vi "Humidity_uncert_2024.vi"(0 "Temperature":dbl=293.15 format="%.4g", 1 "Temperature unit":i32(listbox), 4 "pressure unit":i32(listbox)=1, 5 "Pressure":dbl=100.0 format="%.3f", 6 "Humidity":dbl=50.0 format="%.6f", 7 "humidity unit":i32(listbox)=3) -> (3 "relative humidity":dbl=0.5 format="%.5f", 8 "Psat/p > 1/fe !":bool, 9 "Xw > 1 !":bool, 10 "saturation pressure / Pa":dbl=2339.2491605340156 format="%.1f", 11 "enhanc. factor":dbl=1.0035110316816116 format="%.5g", 12 "DPsat - saturation press. abs. uncert.":dbl=0.23392491605340157 format="%_3f", 13 "xw - molar fraction":dbl=0.011737311692239169, 14 "DPsat/Psat - saturation press. rel. uncert.":dbl=0.0001 format="%.1e", 15 "Def/ef - enhanc. fact. rel. uncert.":dbl=0.00045 format="%.1e", 16 "RH > 1 !":bool, 17 "Def - enhanc. fact. abs. uncert.":dbl=0.0004515799642567252 format="%.6f", 18 "Dxw - molar fraction abs. uncert.":dbl=6.455521430731544e-06 format="%.6f", 19 "Dxw/xw - molar fraction rel. uncert.":dbl=0.00055 format="%.1e")   [LabVIEW 2016]
panel:
  in  "Saturation below 273.16 K":i32(listbox)
  # "±"
  # "±"
  # "±"
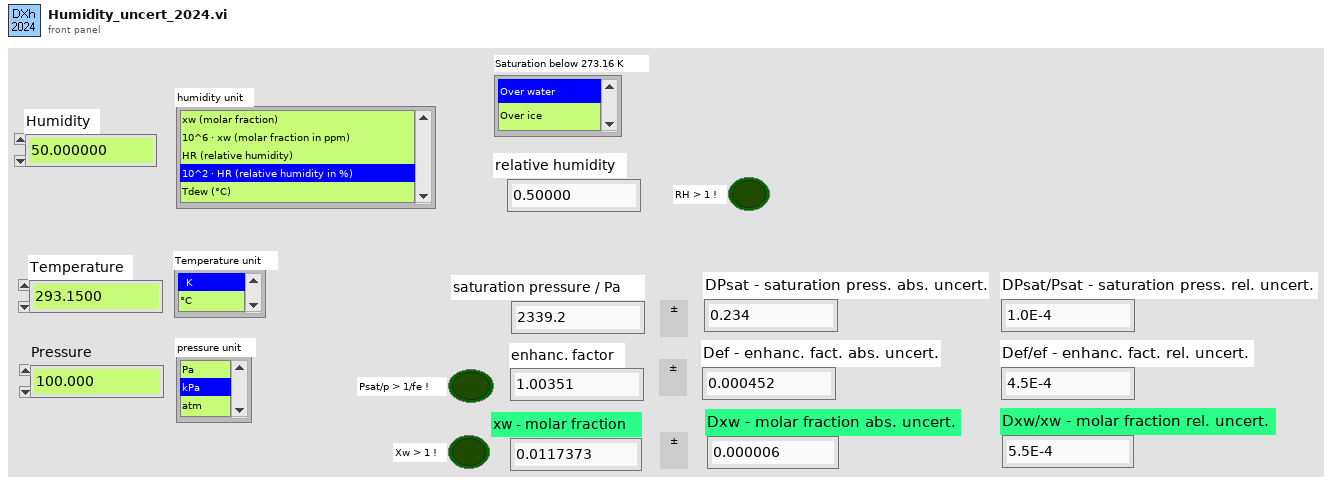
[diagram p1: front panel]
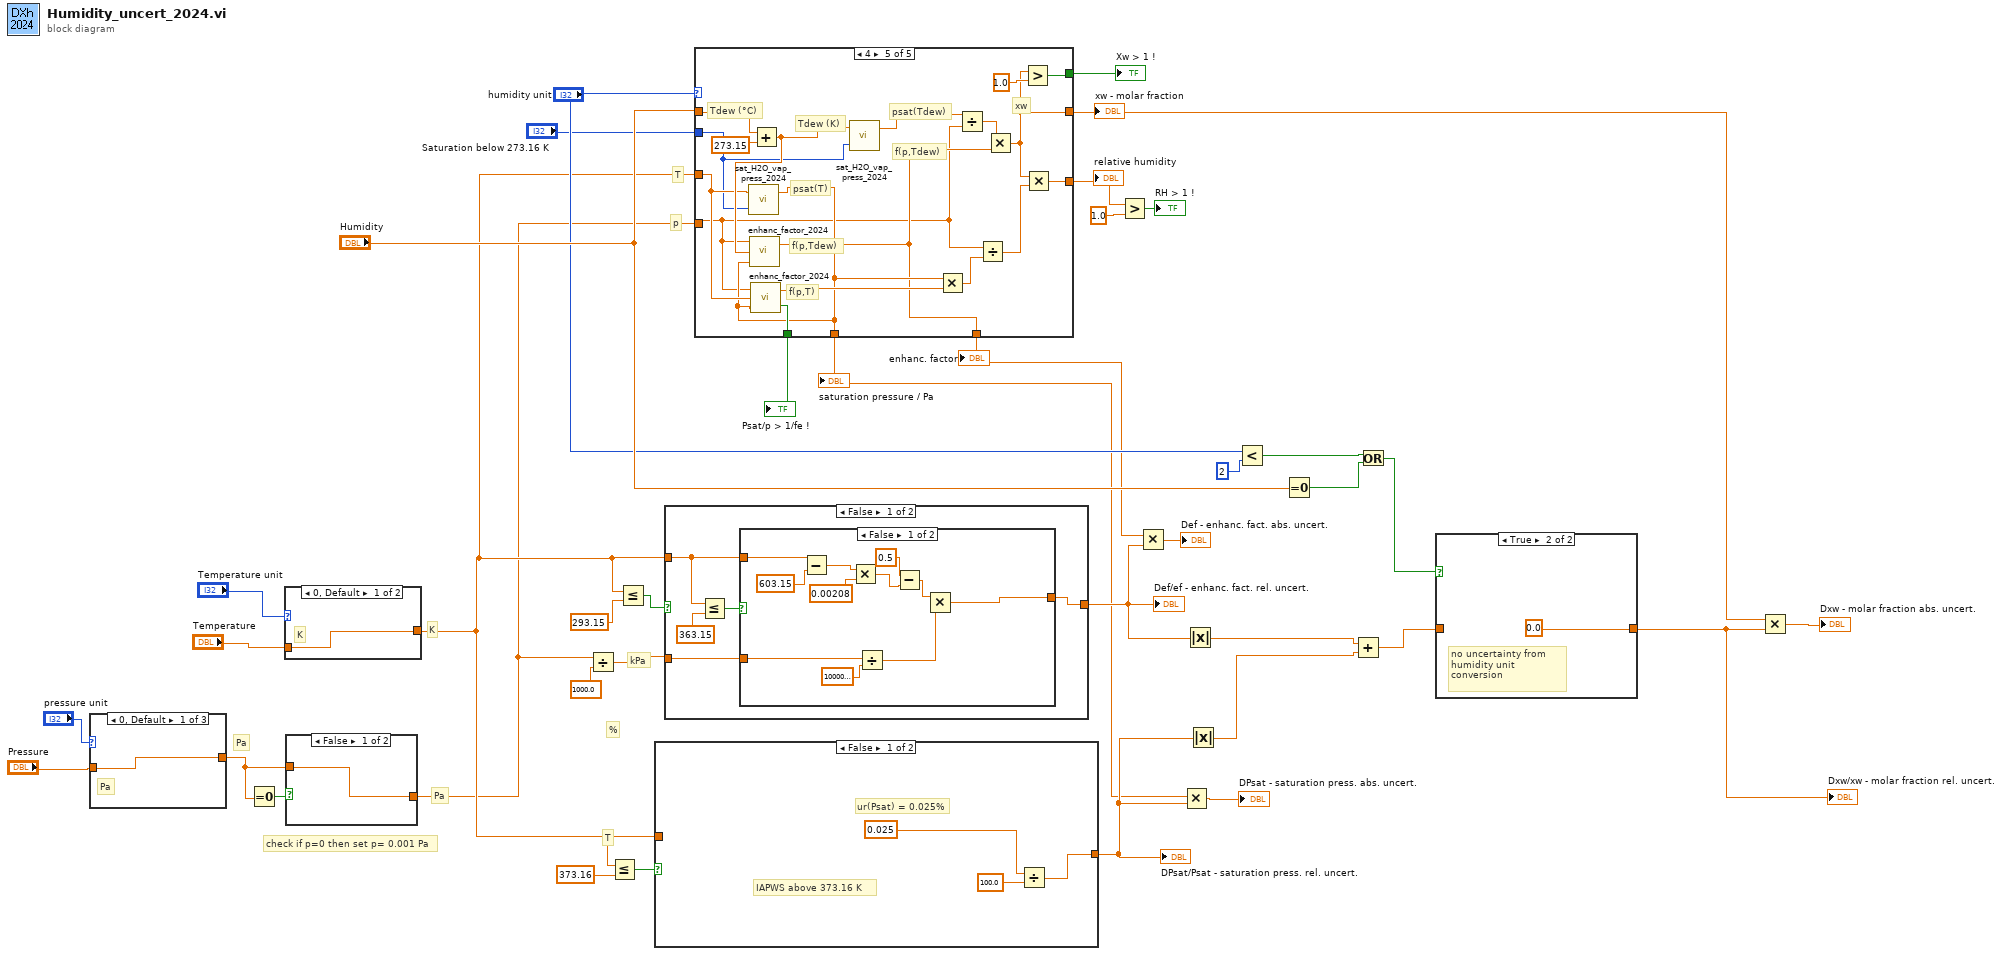
[diagram p0: block diagram]
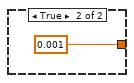
[diagram p2: hidden frame]
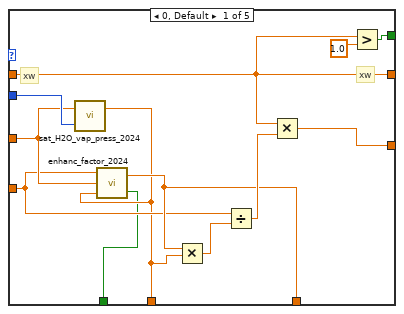
[diagram p3: hidden frame]
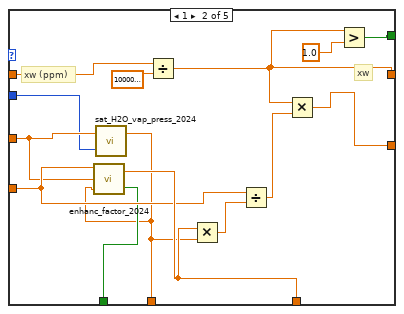
[diagram p4: hidden frame]
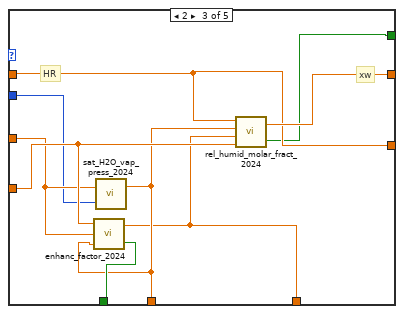
[diagram p5: hidden frame]
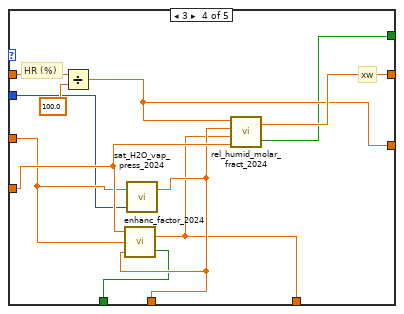
[diagram p6: hidden frame]
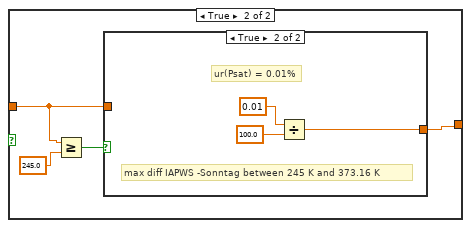
[diagram p8: hidden frame]
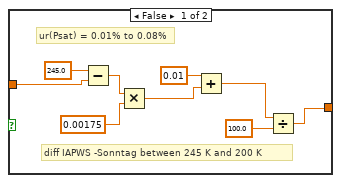
[diagram p9: hidden frame]
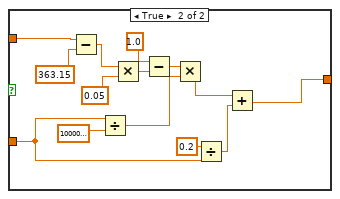
[diagram p10: hidden frame]
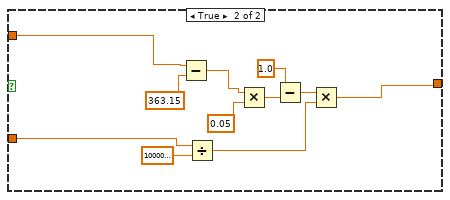
[diagram p11: hidden frame]
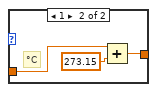
[diagram p12: hidden frame]
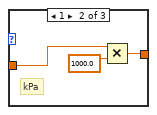
[diagram p13: hidden frame]
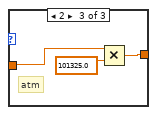
[diagram p14: hidden frame]
diagram:
  # "%"
  # "kPa"
  # "T"
  # "Pa"
  # "check if p=0 then set p= 0.001 Pa"
  # "K"
  # "Pa"
  # "p"
  # "T"
  n1 = case shown="0, Default" "pressure unit" {
    tunnel: [w39 w40 w43] -> w11
    tunnel: "Pressure" -> [w39 w41 w44]
    frame 0, Default {
      # "Pa"
    }
    frame 1 {
      # "kPa"
      n2 = Multiply(x=w41, y=1000.0) -> (x*y=w40:dbl)
    }
    frame 2 {
      # "atm"
      n3 = Multiply(x=w44, y=101325.0) -> (x*y=w43:dbl)
    }
  }
  n4 = Equal To 0?(x=w11) -> (x = 0?=w12:bool)
  n5 = case shown="0, Default" "Temperature unit" {
    tunnel: [w46 w47] -> w7
    tunnel: "Temperature" -> [w46 w48]
    frame 0, Default {
      # "K"
    }
    frame 1 {
      # "°C"
      n6 = Add(x=w48, y=273.15) -> (x+y=w47:dbl)
    }
  }
  n7 = case shown="False" w12 {
    tunnel: [w50 0.001] -> w5
    tunnel: w11 -> [w50 _]
    frame False {
    }
    frame True {
    }
  }
  n8 = Divide(x=w5, y=1000.0) -> (x/y=w4:dbl)
  n9 = Less Or Equal?(x=w7, y=373.16) -> (x <= y?=w32:bool)
  n10 = Less Or Equal?(x=w7, y=293.15) -> (x <= y?=w33:bool)
  n11 = case shown="False" w32 {
    tunnel: [w54 w57] -> w16
    tunnel: w7 -> [_ w55]
    frame False {
      # "ur(Psat) = 0.025%"
      # "IAPWS above 373.16 K"
      n12 = Divide(x=0.025, y=100.0) -> (x/y=w54:dbl)
    }
    frame True {
      n13 = Greater Or Equal?(x=w55, y=245.0) -> (x >= y?=w56:bool)
      n14 = case shown="True" w56 {
        tunnel: [w59 w68] -> w57
        tunnel: w55 -> [w63 _]
        frame False {
          # "ur(Psat) = 0.01% to 0.08%"
          # "diff IAPWS -Sonntag between 245 K and 200 K"
          n15 = Subtract(x=245.0, y=w63) -> (x-y=w62:dbl)
          n16 = Multiply(x=w62, y=0.00175 ("x")) -> (x*y=w61:dbl)
          n17 = Add(x=0.01, y=w61) -> (x+y=w60:dbl)
          n18 = Divide(x=w60, y=100.0) -> (x/y=w59:dbl)
        }
        frame True {
          # "ur(Psat) = 0.01%"
          # "max diff IAPWS -Sonntag between 245 K and 373.16 K"
          n19 = Divide(x=0.01, y=100.0) -> (x/y=w68:dbl)
        }
      }
    }
  }
  "DPsat/Psat - saturation press. rel. uncert." <- w16
  n20 = case shown="False" w33 {
    tunnel: [w71 w101] -> w19
    tunnel: w4 -> [w72 w102]
    tunnel: w7 -> [w73 w111]
    frame False {
      n21 = Less Or Equal?(x=w73, y=363.15) -> (x <= y?=w74:bool)
      n22 = case shown="False" w74 {
        tunnel: w73 -> [w84 w91]
        tunnel: w72 -> [w85 w88]
        tunnel: [w80 w87] -> w71
        frame False {
          n23 = Subtract(x=w84, y=603.15) -> (x-y=w79:dbl)
          n24 = Multiply(x=w79, y=0.00208) -> (x*y=w76:dbl)
          n25 = Divide(x=w85, y=1000000.0) -> (x/y=w82:dbl)
          n26 = Subtract(x=0.5 ("y"), y=w76) -> (x-y=w81:dbl)
          n27 = Multiply(x=w81, y=w82) -> (x*y=w80:dbl)
        }
        frame True {
          n28 = Subtract(x=w91, y=363.15) -> (x-y=w99:dbl)
          n29 = Divide(x=w88, y=1000000.0) -> (x/y=w93:dbl)
          n30 = Multiply(x=w99, y=0.05) -> (x*y=w97:dbl)
          n31 = Subtract(x=1.0, y=w97) -> (x-y=w95:dbl)
          n32 = Multiply(x=w95, y=w93) -> (x*y=w94:dbl)
          n33 = Divide(x=0.2, y=w88) -> (x/y=w89:dbl)
          n34 = Add(x=w94, y=w89) -> (x+y=w87:dbl)
        }
      }
    }
    frame True {
      n35 = Subtract(x=w111, y=363.15) -> (x-y=w109:dbl)
      n36 = Divide(x=w102, y=1000000.0) -> (x/y=w104:dbl)
      n37 = Multiply(x=w109, y=0.05) -> (x*y=w107:dbl)
      n38 = Subtract(x=1.0, y=w107) -> (x-y=w105:dbl)
      n39 = Multiply(x=w105, y=w104) -> (x*y=w101:dbl)
    }
  }
  "Def/ef - enhanc. fact. rel. uncert." <- w19
  n40 = case shown="4" "humidity unit" {
    tunnel: [w113 w125 w145 w157 w159] -> w14
    tunnel: "Humidity" -> [w113 w136 w144 w152 w170]
    tunnel: w5 -> [w117 w132 w146 w155 w162]
    tunnel: w7 -> [w118 w130 w143 w153 w166]
    tunnel: [w116 w127 w140 w150 w164] -> w15
    tunnel: [w119 w133 w139 w147 w163] -> w13
    tunnel: [w121 w131 w144 w154 w171] -> w2
    tunnel: "Saturation below 273.16 K" -> [w120 w129 w142 w148 w161]
    tunnel: [w115 w128 w141 w149 w165] -> w9
    tunnel: [w112 w124 w138 w151 w158] -> w8
    frame 0, Default {
      # "xw"
      # "xw"
      n41 = call "sat_H2O_vap_press_2024.vi"("Saturation below 273.16 K"=w120, "Temperature [K]"=w118) -> ("saturated water vapor pressure [Pa]"=w116:dbl)  [unwired: 1 out]
      n42 = call "enhanc_factor_2024.vi"("saturated vapor pressure [Pa]"=w116, "Temperature / K"=w118, "Pressure / Pa"=w117) -> ("psat/p > 1/fe !"=w115:bool, "enhancement factor"=w119:dbl)
      n43 = Multiply(x=w119, y=w116) -> (x*y=w123:dbl)
      n44 = Divide(x=w117, y=w123) -> (x/y=w122:dbl)
      n45 = Multiply(x=w113, y=w122) -> (x*y=w121:dbl)
      n46 = Greater?(x=w113, y=1.0) -> (0:w112:bool)
    }
    frame 1 {
      # "xw (ppm)"
      # "xw"
      n47 = call "sat_H2O_vap_press_2024.vi"("Saturation below 273.16 K"=w129, "Temperature [K]"=w130) -> ("saturated water vapor pressure [Pa]"=w127:dbl)  [unwired: 1 out]
      n48 = call "enhanc_factor_2024.vi"("saturated vapor pressure [Pa]"=w127, "Temperature / K"=w130, "Pressure / Pa"=w132) -> ("psat/p > 1/fe !"=w128:bool, "enhancement factor"=w133:dbl)
      n49 = Divide(x=w136, y=1000000.0) -> (x/y=w125:dbl)
      n50 = Multiply(x=w133, y=w127) -> (x*y=w135:dbl)
      n51 = Divide(x=w132, y=w135) -> (x/y=w134:dbl)
      n52 = Multiply(x=w125, y=w134) -> (x*y=w131:dbl)
      n53 = Greater?(x=w125, y=1.0) -> (0:w124:bool)
    }
    frame 2 {
      # "xw"
      # "HR"
      n54 = call "sat_H2O_vap_press_2024.vi"("Saturation below 273.16 K"=w142, "Temperature [K]"=w143) -> ("saturated water vapor pressure [Pa]"=w140:dbl)  [unwired: 1 out]
      n55 = call "enhanc_factor_2024.vi"("saturated vapor pressure [Pa]"=w140, "Temperature / K"=w143, "Pressure / Pa"=w146) -> ("psat/p > 1/fe !"=w141:bool, "enhancement factor"=w139:dbl)
      n56 = call "rel_humid_molar_fract_2024.vi"("Pressure [Pa]"=w146, "enhancement factor"=w139, "saturated vapor pressure [Pa]"=w140, "rel. humidity"=w144) -> ("Xw > 1 !"=w138:bool, "xw water mole fraction"=w145:dbl)
    }
    frame 3 {
      # "xw"
      # "HR (%)"
      n57 = Divide(x=w152, y=100.0) -> (x/y=w154:dbl)
      n58 = call "sat_H2O_vap_press_2024.vi"("Saturation below 273.16 K"=w148, "Temperature [K]"=w153) -> ("saturated water vapor pressure [Pa]"=w150:dbl)  [unwired: 1 out]
      n59 = call "enhanc_factor_2024.vi"("saturated vapor pressure [Pa]"=w150, "Temperature / K"=w153, "Pressure / Pa"=w155) -> ("psat/p > 1/fe !"=w149:bool, "enhancement factor"=w147:dbl)
      n60 = call "rel_humid_molar_fract_2024.vi"("Pressure [Pa]"=w155, "enhancement factor"=w147, "saturated vapor pressure [Pa]"=w150, "rel. humidity"=w154) -> ("Xw > 1 !"=w151:bool, "xw water mole fraction"=w157:dbl)
    }
    frame 4 {
      # "f(p,T)"
      # "f(p,Tdew)"
      # "f(p,Tdew)"
      # "psat(Tdew)"
      # "psat(T)"
      # "Tdew (K)"
      # "Tdew (°C)"
      # "xw"
      n61 = call "sat_H2O_vap_press_2024.vi"("Saturation below 273.16 K"=w161, "Temperature [K]"=w166) -> ("saturated water vapor pressure [Pa]"=w164:dbl)  [unwired: 1 out]
      n62 = call "enhanc_factor_2024.vi"("saturated vapor pressure [Pa]"=w164, "Temperature / K"=w166, "Pressure / Pa"=w162) -> ("psat/p > 1/fe !"=w165:bool, "enhancement factor"=w169:dbl)
      n63 = Add(x=w170, y=273.15) -> (x+y=w168:dbl)
      n64 = call "enhanc_factor_2024.vi"("saturated vapor pressure [Pa]"=w164, "Temperature / K"=w168, "Pressure / Pa"=w162) -> ("enhancement factor"=w163:dbl)  [unwired: 1 out]
      n65 = call "sat_H2O_vap_press_2024.vi"("Saturation below 273.16 K"=w161, "Temperature [K]"=w168) -> ("saturated water vapor pressure [Pa]"=w167:dbl)  [unwired: 1 out]
      n66 = Multiply(x=w164, y=w169) -> (x*y=w173:dbl)
      n67 = Divide(x=w167, y=w162) -> (x/y=w174:dbl)
      n68 = Divide(x=w162, y=w173) -> (x/y=w172:dbl)
      n69 = Multiply(x=w174, y=w163) -> (x*y=w159:dbl)
      n70 = Greater?(x=w159, y=1.0) -> (0:w158:bool)
      n71 = Multiply(x=w159, y=w172) -> (x*y=w171:dbl)
    }
  }
  "xw - molar fraction" <- w14
  "saturation pressure / Pa" <- w15
  "enhanc. factor" <- w13
  "relative humidity" <- w2
  "Psat/p > 1/fe !" <- w9
  "Xw > 1 !" <- w8
  n72 = Greater?(x=w2, y=1.0) -> (0:→"RH > 1 !":bool)
  n73 = Multiply(x=w13, y=w19) -> (x*y=→"Def - enhanc. fact. abs. uncert.":dbl)
  n74 = Multiply(x=w15, y=w16) -> (x*y=→"DPsat - saturation press. abs. uncert.":dbl)
  n75 = Absolute Value(x=w19) -> (abs(x)=w30:dbl)
  n76 = Absolute Value(x=w16) -> (abs(x)=w29:dbl)
  n77 = Less?(x="humidity unit", y=2) -> (x < y?=w26:bool)
  n78 = Equal To 0?(x="Humidity") -> (x = 0?=w25:bool)
  n79 = Add(x=w30, y=w29) -> (x+y=w28:dbl)
  n80 = Or(x=w26, y=w25) -> (x .or. y?=w24:bool)
  n81 = case shown="True" w24 {
    tunnel: w28 -> [w176 _]
    tunnel: [w176 0.0] -> w22
    frame False {
    }
    frame True {
      # "no uncertainty from humidity unit conversion"
    }
  }
  "Dxw/xw - molar fraction rel. uncert." <- w22
  n82 = Multiply(x=w14, y=w22) -> (x*y=→"Dxw - molar fraction abs. uncert.":dbl)
